vi "Configure_PSG_ Frequency_Power_bool.vi"(3 "Attenuator Auto Mode (T:Enable)":bool=TRUE, 5 "Attenuator Auto Mode (T:Enable) 2":bool=TRUE) -> ()   [LabVIEW 2011]
doc: "This example shows how to configure the frequency and power of the output signal."
uses:
  <instrlib>/Agilent PSG MXG Series/Agilent PSG MXG Series.lvlib
panel:
  in  "VISA resource name":refnum<visa-resource-name>
  in  "ALC Level (1 dB)":dbl=1.0
  in  "Power (-130 dBm)":dbl=-130.0
  in  "Frequency (100 kHz)":dbl=100000.0
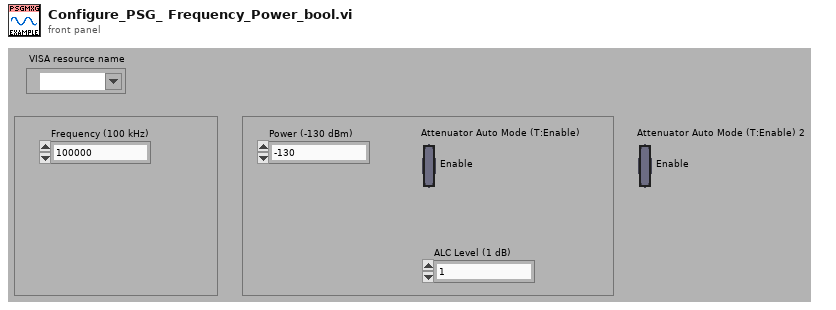
[diagram p1: front panel]
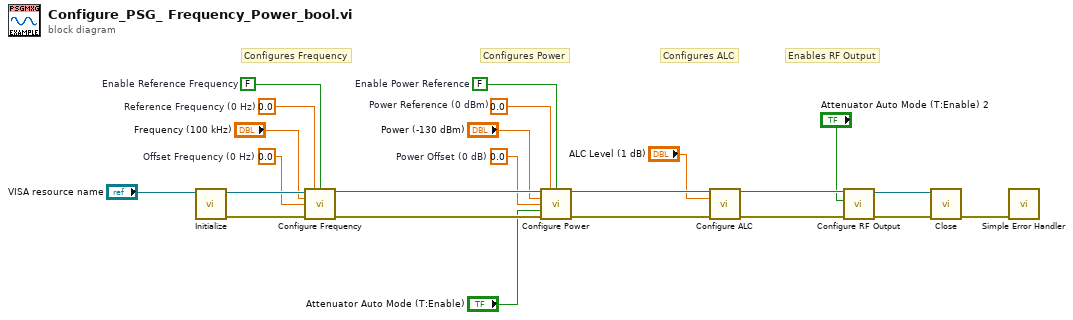
[diagram p0: block diagram]
diagram:
  w6 = 0.0  # Offset Frequency (0 Hz)
  w7 = 0.0  # Reference Frequency (0 Hz)
  w4 = 0.0  # Power Reference (0 dBm)
  w3 = 0.0  # Power Offset (0 dB)
  w5 = FALSE  # Enable Power Reference
  w8 = FALSE  # Enable Reference Frequency
  # "Enables RF Output"
  # "Configures ALC"
  # "Configures Power"
  # "Configures Frequency"
  n1 = call <instrlib>:"Initialize.vi"("VISA resource name"="VISA resource name") -> ("error out"=w22:errorcluster, "VISA resource name out"=w23:refnum<visa-resource-name>)  [unwired: 9 in]
  n2 = call <instrlib>:"Configure Frequency.vi"("VISA resource name"=w23, "Reference Frequency (0 Hz)"=w7, "Enable Reference Frequency (F:Disable)"=w8, "Frequency (100 kHz)"="Frequency (100 kHz)", "Offset Frequency (0 Hz)"=w6, "error in (no error)"=w22) -> ("VISA resource name out"=w21:refnum<visa-resource-name>, "error out"=w20:errorcluster)  [unwired: 8 in]
  n3 = call <instrlib>:"Configure Power.vi"("VISA resource name"=w21, "Power Reference (0 dBm)"=w4, "Enable Power Reference (F:Disable)"=w5, "Power (-130 dBm)"="Power (-130 dBm)", "Power Offset (0 dB)"=w3, "Attenuator Auto Mode (T:Enable)"="Attenuator Auto Mode (T:Enable)", "error in (no error)"=w20) -> ("VISA resource name out"=w19:refnum<visa-resource-name>, "error out"=w18:errorcluster)  [unwired: 7 in]
  n4 = call <instrlib>:"Configure ALC.vi"("VISA resource name"=w19, "ALC Level (1 dB)"="ALC Level (1 dB)", "error in (no error)"=w18) -> ("VISA resource name out"=w16:refnum<visa-resource-name>, "error out"=w15:errorcluster)  [unwired: 11 in]
  n5 = call <instrlib>:"Configure RF Output.vi"("error in (no error)"=w15, "Enable RF Output (F:Disable)"="Attenuator Auto Mode (T:Enable) 2", "VISA resource name"=w16) -> ("error out"=w13:errorcluster, "VISA resource name out"=w14:refnum<visa-resource-name>)  [unwired: 7 in]
  n6 = call <instrlib>:"Close.vi"("error in (no error)"=w13, "VISA resource name"=w14) -> ("error out"=w17:errorcluster)  [unwired: 9 in]
  n7 = call <vilib>:"Simple Error Handler.vi"("error in (no error)"=w17) -> ()  [unwired: 4 in, 5 out]
